vi "xmlProtocol1.vi"(10 "Array":string[](array[string]), 11 "Numeric":i32) -> ()   [LabVIEW 2018]
uses:
  Global Variables.vi
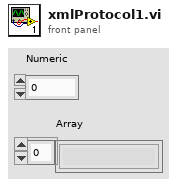
[diagram p1: front panel]
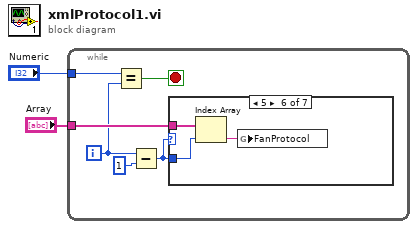
[diagram p0: block diagram]
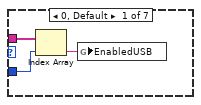
[diagram p2: hidden frame]
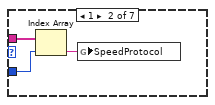
[diagram p3: hidden frame]
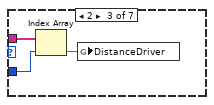
[diagram p4: hidden frame]
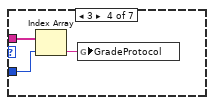
[diagram p5: hidden frame]
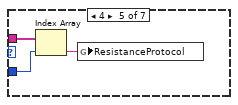
[diagram p6: hidden frame]
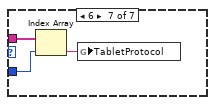
[diagram p7: hidden frame]
diagram:
  n1 = while {
    tunnel: "Array" -> [w8]
    tunnel: "Numeric" -> [w6]
    i -> [w4]
    stop <- w7 stop-if-true
    n2 = Equal?(x=w6, y=w4) -> (x = y?=w7:bool)
    n3 = Subtract(x=w4, y=1) -> (x-y=w5:i32)
    n4 = case shown="5" w5 {
      tunnel: w8 -> [w11 w14 w17 w20 w23 w26 w29]
      tunnel: w5 -> [w10 w13 w16 w19 w22 w25 w28]
      frame 0, Default {
        n5 = Index Array(array=w11, index=w10) -> (element=w9:string)
        n6 = global write "Global Variables.vi" "EnabledUSB"(w9) -> ()
      }
      frame 1 {
        n7 = Index Array(array=w14, index=w13) -> (element=w12:string)
        n8 = global write "Global Variables.vi" "SpeedProtocol"(w12) -> ()
      }
      frame 2 {
        n9 = Index Array(array=w17, index=w16) -> (element=w15:string)
        n10 = global write "Global Variables.vi" "DistanceDriver"(w15) -> ()
      }
      frame 3 {
        n11 = Index Array(array=w20, index=w19) -> (element=w18:string)
        n12 = global write "Global Variables.vi" "GradeProtocol"(w18) -> ()
      }
      frame 4 {
        n13 = Index Array(array=w23, index=w22) -> (element=w21:string)
        n14 = global write "Global Variables.vi" "ResistanceProtocol"(w21) -> ()
      }
      frame 5 {
        n15 = Index Array(array=w26, index=w25) -> (element=w24:string)
        n16 = global write "Global Variables.vi" "FanProtocol"(w24) -> ()
      }
      frame 6 {
        n17 = Index Array(array=w29, index=w28) -> (element=w27:string)
        n18 = global write "Global Variables.vi" "TabletProtocol"(w27) -> ()
      }
    }
  }
